vi "Determine Failure Action.vi"(8 "error in (no error)":errorcluster, 10 "Failure Action Change Event References":T1, 11 "Assert Message in":T2) -> (0 "error out":errorcluster, 3 "Assert Message out":T2)   [LabVIEW 2016, in "Assert API Components.lvlib" / "Log Assert Core.lvlib"]
uses:
  Log Assert Core.lvlib
  Message Data.ctl
  Failure Actions.ctl
  VI References.ctl
  Failure Action Change Event Reference.ctl
  Assert API Components.lvlib
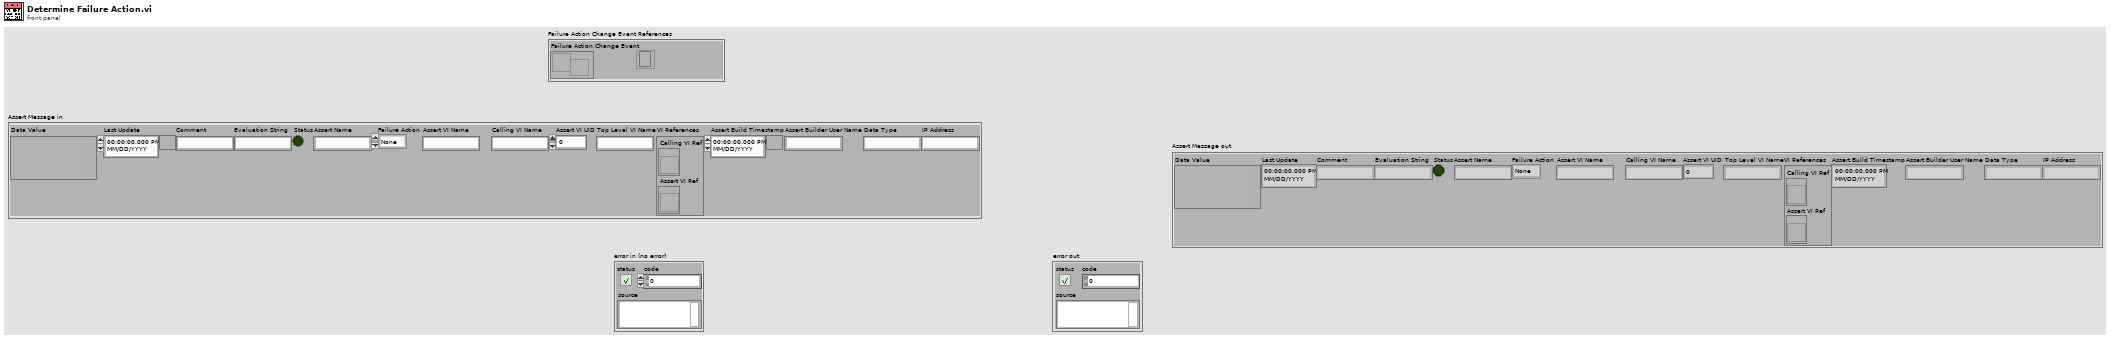
[diagram p1: front panel]
types:
  T1 = typedef "Assert API Components.lvlib/Log Assert Core.lvlib/Failure Action Change Event Reference.ctl" = cluster{"Failure Action Change Event":refnum<user-event>, "Event Registration Refnum":refnum<event-registration>}
  T2 = typedef "Assert API Components.lvlib/Message Data.ctl" = cluster{"Data Value":variant, "Last Update":timestamp, "Comment":string, "Evaluation String":string, "Status":bool, "Assert Name":string, "Failure Action":T3, "Assert VI Name":string, "Calling VI Name":string, "Assert VI UID":i32, "Top Level VI Name":string, "VI References":T4, "Assert Build Timestamp":timestamp, "Assert Builder User Name":string, "Data Type":string, "IP Address":string}
  T3 = typedef "Assert API Components.lvlib/Failure Actions.ctl" = enum16{"None", "Log To File", "Pause Execution", "Abort Execution"}
  T4 = typedef "Assert API Components.lvlib/VI References.ctl" = cluster{"Calling VI Ref":refnum<vi>, "Assert VI Ref":refnum<vi>}
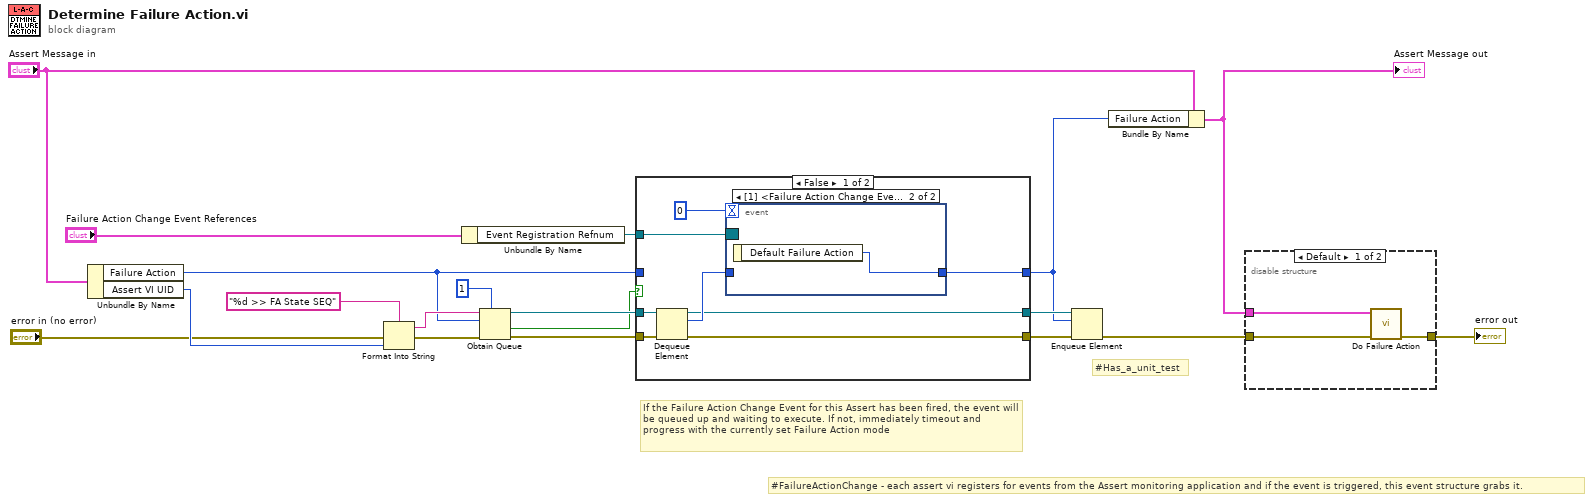
[diagram p0: block diagram]
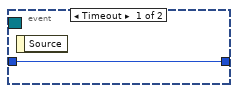
[diagram p3: hidden frame]
diagram:
  # "#Has_a_unit_test"
  # "#FailureActionChange - each assert vi registers for events from the Assert monitoring application and if the event is triggered, this event structure grabs it."
  # "If the Failure Action Change Event for this Assert has been fired, the event will be queued up and waiting to execute. If not, immediately timeout and progress with the currently set Failure Action mode"
  n1 = Unbundle By Name("Assert Message in") -> ("Failure Action"=w4:T3, "Assert VI UID"=w10:i32)
  n2 = Format Into String(format string="%d >> FA State SEQ" ("string"), error in="error in (no error)", w10) -> (resulting string=w11:string, error out=w9:errorcluster)  [unwired: 1 in]
  n3 = Unbundle By Name("Failure Action Change Event References") -> ("Event Registration Refnum"=w17:refnum<event-registration>)
  n4 = Obtain Queue(max queue size (-1, unlimited)=1, name (unnamed)=w11, element data type=w4, error in (no error)=w9) -> (queue out=w6:refnum<queue>, created new?=w5:bool, error out=w8:errorcluster)  [unwired: 1 in]
  n5 = case shown="False" w5 {
    tunnel: [w25 w32] -> w3
    tunnel: w17 -> [w26 _]
    tunnel: [w23 w30] -> w19
    tunnel: [w22 w31] -> w18
    tunnel: w4 -> [_ w32]
    tunnel: w8 -> [w21 w30]
    tunnel: w6 -> [w20 w31]
    frame False {
      n6 = Dequeue Element(queue=w20, error in (no error)=w21) -> (queue out=w22:refnum<queue>, element=w24:T3, error out=w23:errorcluster)  [unwired: 1 in, 1 out]
      n7 = event shown="[1] <Failure Action Change Event>: User Event" {
        selector: w26 -> [_ _]
        dyn-events: _ -> [_ _]
        timeout: 0 -> [_ _]
        tunnel: [w28 w29] -> w25
        tunnel: w24 -> [w28 _]
        event Timeout {
          n8 = event-data() -> ()  [unwired: 1 in, 1 out]
        }
        event User Event {
          n9 = event-data() -> ("Default Failure Action"=w29:T3)  [unwired: 1 in]
        }
      }
    }
    frame True {
      # "Takes the default failure action on the first call but thereafter looks in the SEQ"
    }
  }
  n10 = Enqueue Element(queue=w18, element=w3, error in (no error)=w19) -> (error out=w2:errorcluster)  [unwired: 1 in, 2 out]
  n11 = Bundle By Name(cluster="Assert Message in", "Failure Action"=w3) -> (w15:T2)
  "Assert Message out" <- w15
  n12 = disable-structure shown="Default" {
    disable-tunnel: w15 -> [w35 _]
    disable-tunnel: w2 -> [w34 w36]
    disable-tunnel: [w33 w36] -> w1
    frame condition #0 (active) {
      n13 = call "Do Failure Action.vi"("error in (no error)"=w34, "Assert Message in"=w35) -> ("error out"=w33:errorcluster)  [unwired: 9 in]
    }
    frame condition #1 {
      # "Do not perform the failure action when doing a #UnitTest"
    }
  }
  "error out" <- w1
